vi "Anaolg OUT LED.vi"() -> ()   [LabVIEW 2014]
uses:
  <vilib>/DAQmx/create/channels.llb/DAQmx Create Channel (AO-Voltage-Basic).vi
  <vilib>/DAQmx/write.llb/DAQmx Write (Analog DBL 1Chan 1Samp).vi
panel:
  out "error out":errorcluster
  in  "Voltage Out":dbl(slide) min=0.0 max=10.0 step=0.01 scale=0.0..10.0
  in  "Turn ON":bool
  in  "physical channel":tag="Dev1/ao0"
  in  "stop":bool
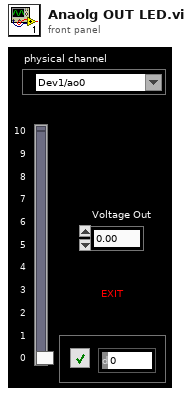
[diagram p1: front panel]
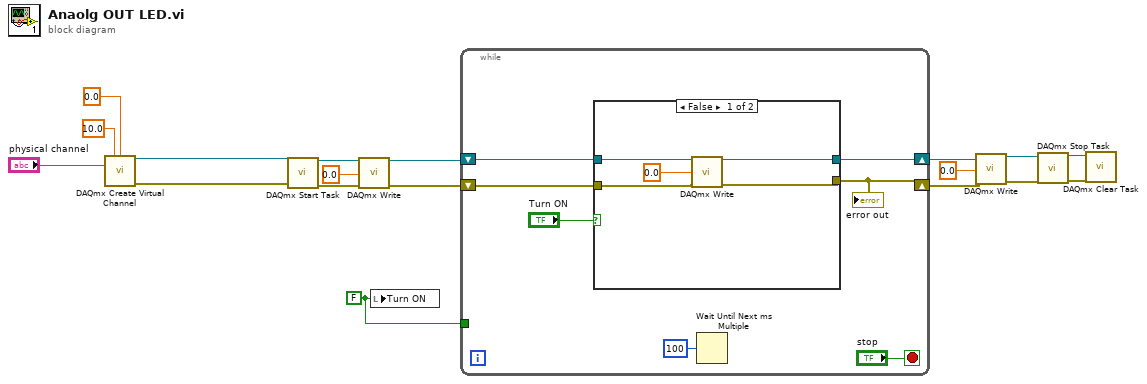
[diagram p0: block diagram]
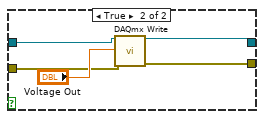
[diagram p2: hidden frame]
diagram:
  w1 = FALSE ("Turn ON")
  n1 = call-poly <vilib>:"DAQmx Create Virtual Channel.vi"("maximum value"=10.0, "minimum value"=0.0, "physical channels"="physical channel") -> ("task out"=w3:refnum<k21>, "error out"=w2:errorcluster)  [unwired: 11 in]
  n2 = call <vilib>:"DAQmx Start Task.vi"("task/channels in"=w3, "error in"=w2) -> ("task out"=w15:refnum<k21>, "error out"=w8:errorcluster)  [unwired: 12 in]
  n3 = call-poly <vilib>:"DAQmx Write.vi"("task/channels in"=w15, "data"=0.0, "error in"=w8) -> ("task out"=w14:refnum<k21>, "error out"=w7:errorcluster)  [unwired: 10 in, 1 out]
  n4 = local write "Turn ON"(w1) -> ()
  n5 = while {
    shift-right: [w22] -> w11
    shift-left: w14 -> [w23]
    shift-right: [w19] -> w6
    shift-left: w7 -> [w20]
    tunnel: w1 -> [_]
    stop <- "stop" stop-if-true
    n6 = case shown="False" "Turn ON" {
      tunnel: [w29 w34] -> w22
      tunnel: w23 -> [w30 w35]
      tunnel: w20 -> [w26 w32]
      tunnel: [w28 w31] -> w19
      frame False {
        n7 = call-poly <vilib>:"DAQmx Write.vi"("task/channels in"=w30, "data"=0.0, "error in"=w26) -> ("task out"=w29:refnum<k21>, "error out"=w28:errorcluster)  [unwired: 10 in, 1 out]
      }
      frame True {
        n8 = call-poly <vilib>:"DAQmx Write.vi"("task/channels in"=w35, "data"="Voltage Out", "error in"=w32) -> ("task out"=w34:refnum<k21>, "error out"=w31:errorcluster)  [unwired: 10 in, 1 out]
      }
    }
    "error out" <- w19
    n9 = Wait Until Next ms Multiple(millisecond multiple=u32 100) -> ()  [unwired: 1 out]
  }
  n10 = call-poly <vilib>:"DAQmx Write.vi"("task/channels in"=w11, "data"=0.0, "error in"=w6) -> ("task out"=w10:refnum<k21>, "error out"=w5:errorcluster)  [unwired: 10 in, 1 out]
  n11 = call <vilib>:"DAQmx Stop Task.vi"("task/channels in"=w10, "error in"=w5) -> ("task out"=w9:refnum<k21>, "error out"=w4:errorcluster)  [unwired: 12 in]
  n12 = call <vilib>:"DAQmx Clear Task.vi"("task in"=w9, "error in"=w4) -> ()  [unwired: 13 in, 1 out]
